vi "경과시간.vi"() -> ()   [LabVIEW 2014]
panel:
  out "T":dbl
  out "웨이브폼 차트":dbl(graph)
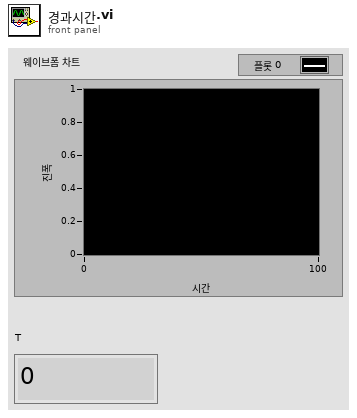
[diagram p1: front panel]
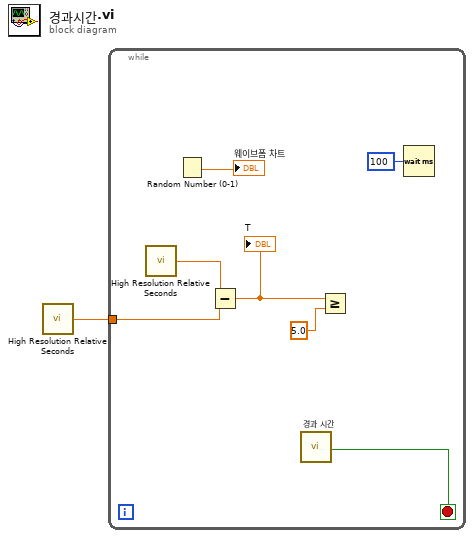
[diagram p0: block diagram]
diagram:
  n1 = call <vilib>:"High Resolution Relative Seconds.vi"() -> ("relative seconds"=w1:dbl)
  n2 = while {
    tunnel: w1 -> [w5]
    stop <- w2 stop-if-true
    n3 = call <vilib>:"High Resolution Relative Seconds.vi"() -> ("relative seconds"=w6:dbl)
    n4 = Random Number (0-1)() -> (number: 0 to 1=→"웨이브폼 차트":dbl)
    n5 = Subtract(x=w6, y=w5) -> (x-y=w4:dbl)
    "T" <- w4
    n6 = call "경과 시간"() -> ("Time has Elapsed"=w2:bool)  [unwired: 12 in, 7 out]
    n7 = Greater Or Equal?(x=w4, y=5.0) -> ()  [unwired: 1 out]
    n8 = Wait (ms)(milliseconds to wait=u32 100 ("대기 시간(ms)")) -> ()  [unwired: 1 out]
  }
